vi "EOL Digital Outputs v3.vi"(7 "task/channels in":refnum<k21> caption="DO Task", 8 "Error In":errorcluster, 9 "DO Status":T1[](array[typedef]), 11 "Mode":T3(ring)) -> (0 "Error Out":errorcluster, 2 "Digital Out State 1":bool[](array[boolean]))   [LabVIEW 2018]
uses:
  05.UserVI's/type defs/EOL Global Digital Output Cluster Control.ctl
  05.UserVI's/type defs/EOL Global Digital Output Control.ctl
  <vilib>/DAQmx/write.llb/DAQmx Write (Digital 1D Bool NChan 1Samp 1Line).vi
  <vilib>/DAQmx/read.llb/DAQmx Read (Digital 1D Bool NChan 1Samp 1Line).vi
  <vilib>/DAQmx/miscellaneous.llb/DAQmx Fill In Error Info.vi
  <resource>/objmgr/daqmx.rc
panel:
  out "NumChans":u32
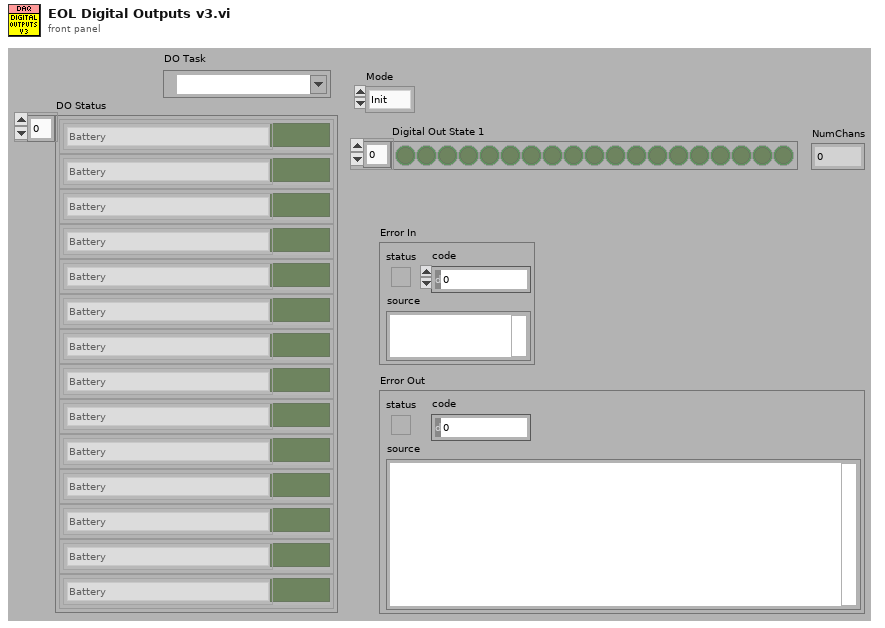
[diagram p1: front panel]
types:
  T1 = typedef "EOL Global Digital Output Cluster Control.ctl" = cluster{"Status":bool, "Global DO Ch":T2}
  T2 = typedef "EOL Global Digital Output Control.ctl" = enum16{"Battery", "IGN High", "IGN Low", "LIN", "CAN", "Switch 1", "Switch 2", "Switch 3", "Switch 4", "Switch 5", "Switch 6", "Glass Analog Switch 1", "Glass Analog Switch 2", "Glass Analog Switch 3", "Glass Analog Switch 4", "Sunshade Analog Switch 1", "Sunshade Analog Switch 2", "Sunshade Analog Switch 3", "Sunshade Analog Switch 4", "Glass Motor Relay 1", "Glass Motor Relay 2", "Sunshade Motor Relay 1", "Sunshade Motor Relay 2"}
  T3 = enum16{"Init", "Write", "Write All", "Clear All", "Stop", "Read"}
  T4 = cluster{"Digital Out State 1":bool[], "Error":errorcluster}
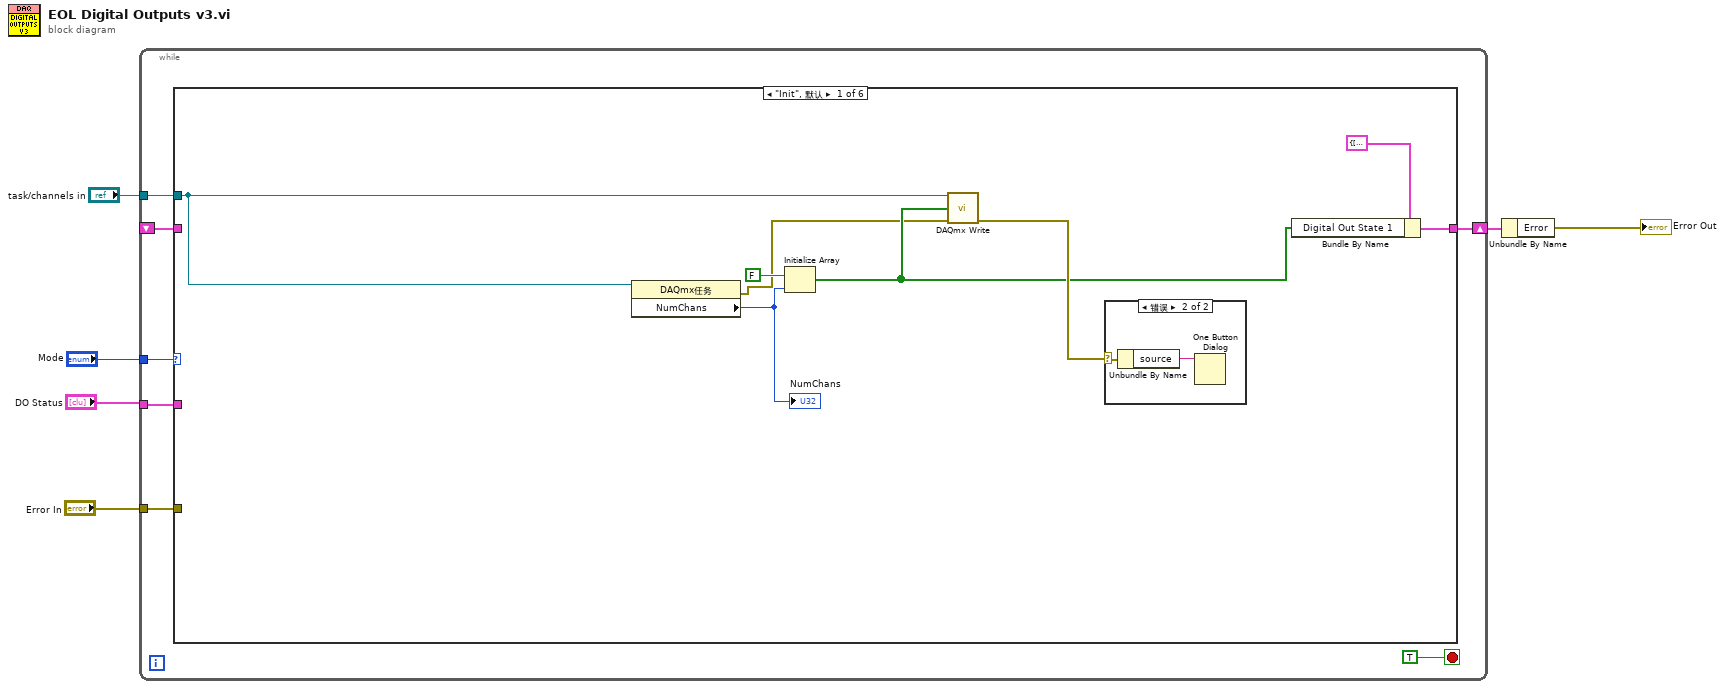
[diagram p0: block diagram]
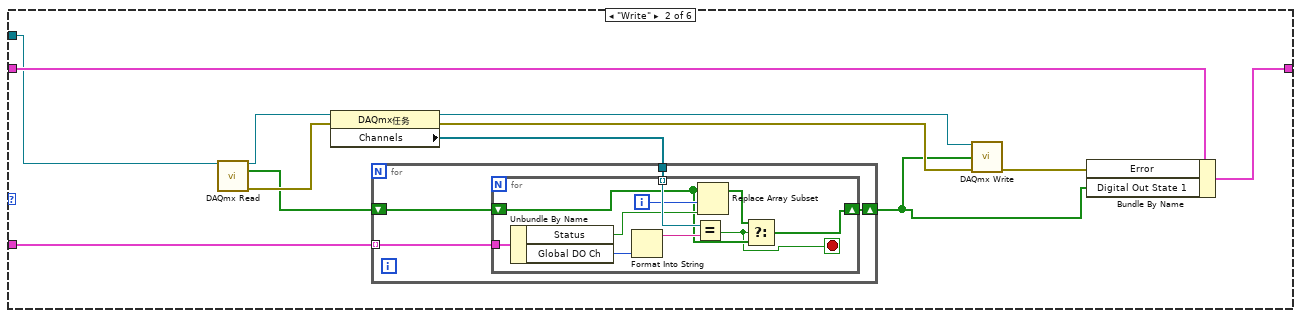
[diagram p3: hidden frame]
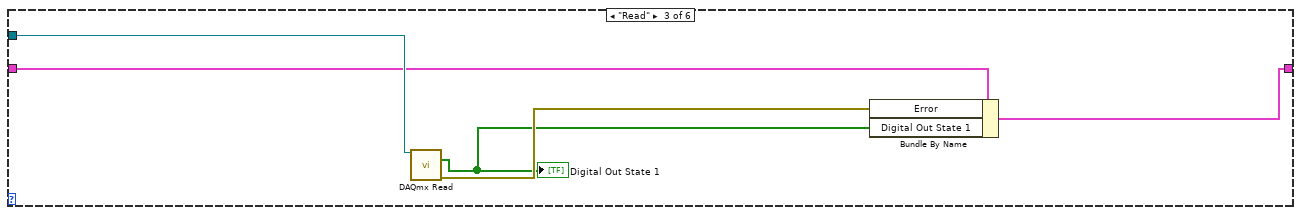
[diagram p4: hidden frame]
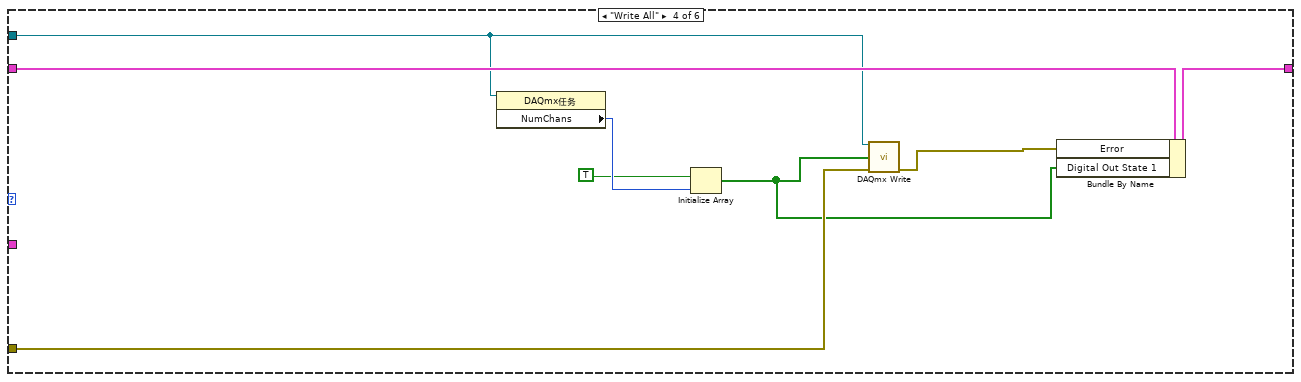
[diagram p5: hidden frame]
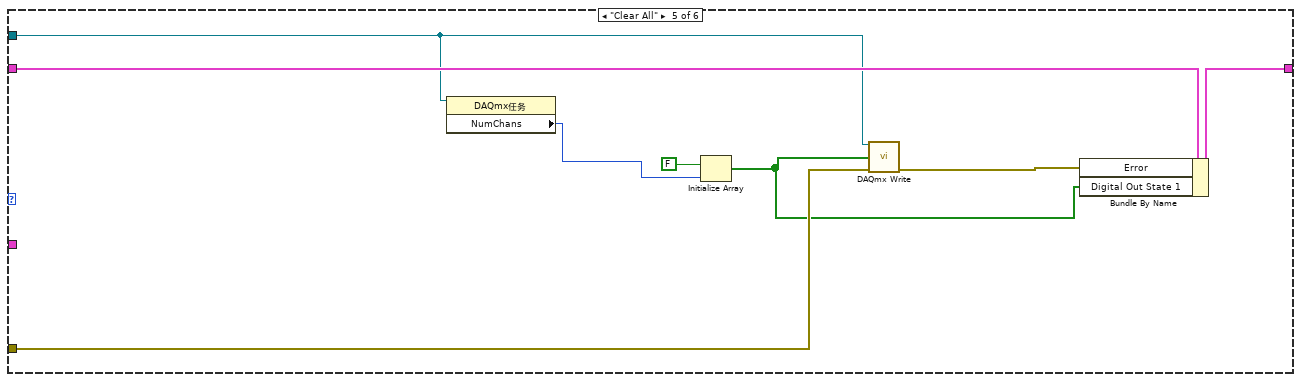
[diagram p6: hidden frame]
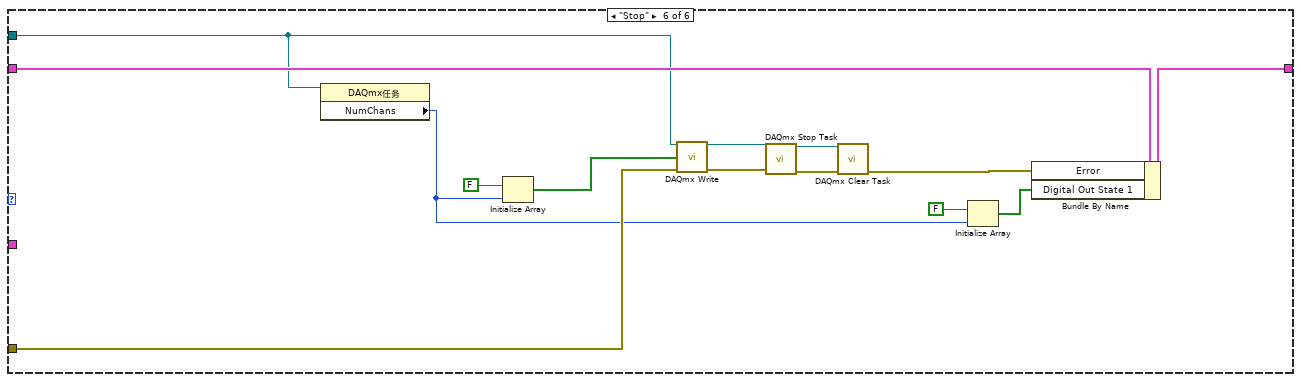
[diagram p7: hidden frame]
diagram:
  n1 = while {
    tunnel: "Mode" -> [w12]
    shift-right: [w11] -> w4
    shift-left: _ -> [w10]
    tunnel: "DO Status" -> [w9]
    tunnel: "Error In" -> [w8]
    tunnel: "task/channels in" -> [w7]
    stop <- TRUE stop-if-true
    n2 = case shown="\"Init\", 默认" w12 {
      tunnel: [w20 w34 w51 w61 w69 w83] -> w11
      tunnel: w10 -> [_ w35 w53 w62 w70 w84]
      tunnel: w9 -> [_ w31 _ _ _ _]
      tunnel: w8 -> [_ _ _ w59 w66 w79]
      tunnel: w7 -> [w17 w29 w54 w57 w64 w72]
      frame "Init", Default {
        n3 = property class="DAQmx任务"(reference=w17) -> (error out=w15:errorcluster, "NumChans"=w14:u32)  [unwired: 1 in, 1 out]
        "NumChans" <- w14
        n4 = Initialize Array(FALSE, w14) -> (w16:bool[])
        n5 = call-poly <vilib>:"DAQmx Write.vi"("task/channels in"=w17, "data"=w16, "error in"=w15) -> ("error out"=w19:errorcluster)  [unwired: 10 in, 2 out]
        n6 = case shown="错误" w19 {
          selector: w19 -> [_ w23]
          frame No Error {
          }
          frame Error {
            n7 = Unbundle By Name(w23) -> ("source"=w22:string)
            n8 = One Button Dialog(message=w22) -> ()  [unwired: 1 in, 1 out]
          }
        }
        n9 = Bundle By Name(cluster=T4 {"Digital Out State 1"=[], "Error"={"status"=FALSE, "code"=0, "source"=""}}, "Digital Out State 1"=w16) -> (w20:T4)
      }
      frame "Write" {
        n10 = call-poly <vilib>:"DAQmx Read.vi"("task/channels in"=w29) -> ("task out"=w28:refnum<k21>, "data"=w25:bool[], "error out"=w27:errorcluster)  [unwired: 12 in]
        n11 = property class="DAQmx任务"(reference=w28, error in=w27) -> (reference out=w32:refnum<k21>, error out=w26:errorcluster, "Channels"=w30:refnum<k21>[])
        n12 = for {
          tunnel: w31 -> [w39] mode=indexing
          tunnel: w30 -> [w38]
          shift-right: [w36] -> w24
          shift-left: w25 -> [w37]
          n13 = for {
            tunnel: w39 -> [w49]
            tunnel: w38 -> [w47] mode=indexing
            shift-right: [w41] -> w36
            shift-left: w37 -> [w42]
            i -> [w45]
            stop <- w40 stop-if-true
            n14 = Unbundle By Name(w49) -> ("Status"=w44:bool, "Global DO Ch"=w48:T2)
            n15 = Format Into String(w48) -> (resulting string=w46:string)  [unwired: 3 in, 1 out]
            n16 = Equal?(x=w47, y=w46) -> (x = y?=w40:bool)
            n17 = Replace Array Subset(array=w42, new element=w44, index=w45) -> (w43:bool[])
            n18 = Select(t=w43, s=w40, f=w42) -> (s? t:f=w41:bool[])
          }
        }
        n19 = call-poly <vilib>:"DAQmx Write.vi"("task/channels in"=w32, "data"=w24, "error in"=w26) -> ("error out"=w33:errorcluster)  [unwired: 10 in, 2 out]
        n20 = Bundle By Name(cluster=w35, "Error"=w33, "Digital Out State 1"=w24) -> (w34:T4)
      }
      frame "Read" {
        n21 = call-poly <vilib>:"DAQmx Read.vi"("task/channels in"=w54) -> ("data"=w50:bool[], "error out"=w52:errorcluster)  [unwired: 12 in, 1 out]
        "Digital Out State 1" <- w50
        n22 = Bundle By Name(cluster=w53, "Error"=w52, "Digital Out State 1"=w50) -> (w51:T4)
      }
      frame "Write All" {
        n23 = property class="DAQmx任务"(reference=w57) -> ("NumChans"=w56:u32)  [unwired: 1 in, 2 out]
        n24 = Initialize Array(TRUE, w56) -> (w58:bool[])
        n25 = call-poly <vilib>:"DAQmx Write.vi"("task/channels in"=w57, "data"=w58, "error in"=w59) -> ("error out"=w60:errorcluster)  [unwired: 10 in, 2 out]
        n26 = Bundle By Name(cluster=w62, "Error"=w60, "Digital Out State 1"=w58) -> (w61:T4)
      }
      frame "Clear All" {
        n27 = property class="DAQmx任务"(reference=w64) -> ("NumChans"=w63:u32)  [unwired: 1 in, 2 out]
        n28 = Initialize Array(FALSE, w63) -> (w65:bool[])
        n29 = call-poly <vilib>:"DAQmx Write.vi"("task/channels in"=w64, "data"=w65, "error in"=w66) -> ("error out"=w68:errorcluster)  [unwired: 10 in, 2 out]
        n30 = Bundle By Name(cluster=w70, "Error"=w68, "Digital Out State 1"=w65) -> (w69:T4)
      }
      frame "Stop" {
        n31 = property class="DAQmx任务"(reference=w72) -> ("NumChans"=w71:u32)  [unwired: 1 in, 2 out]
        n32 = Initialize Array(FALSE, w71) -> (w80:bool[])
        n33 = call-poly <vilib>:"DAQmx Write.vi"("task/channels in"=w72, "data"=w80, "error in"=w79) -> ("task out"=w76:refnum<k21>, "error out"=w74:errorcluster)  [unwired: 10 in, 1 out]
        n34 = call <vilib>:"DAQmx Stop Task.vi"("task/channels in"=w76, "error in"=w74) -> ("task out"=w75:refnum<k21>, "error out"=w73:errorcluster)  [unwired: 12 in]
        n35 = call <vilib>:"DAQmx Clear Task.vi"("task in"=w75, "error in"=w73) -> ("error out"=w82:errorcluster)  [unwired: 13 in]
        n36 = Initialize Array(FALSE, w71) -> (w77:bool[])
        n37 = Bundle By Name(cluster=w84, "Error"=w82, "Digital Out State 1"=w77) -> (w83:T4)
      }
    }
  }
  n38 = Unbundle By Name(w4) -> ("Error"=→"Error Out":errorcluster)
